vi "Base.vi"(11 "Boolean IN":bool) -> (3 "Boolean OUT":bool)   [LabVIEW 2025]
uses:
  <vilib>/JDP Science/JDP Science Common Utilities/JDP Utility.lvlib
panel:
  in  "Array":void[](array[numeric])
  in  "Multicolumn Listbox":i32(listbox)
  out "XY Graph":cluster{"X":dbl, "Y":dbl}[](graph)
  in  "Tree":string(tree)
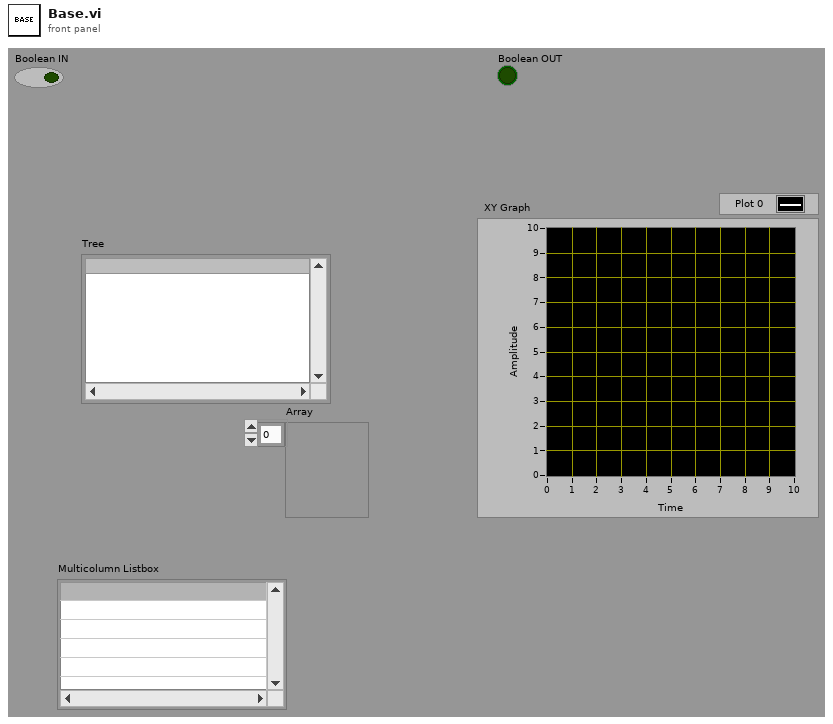
[diagram p1: front panel]
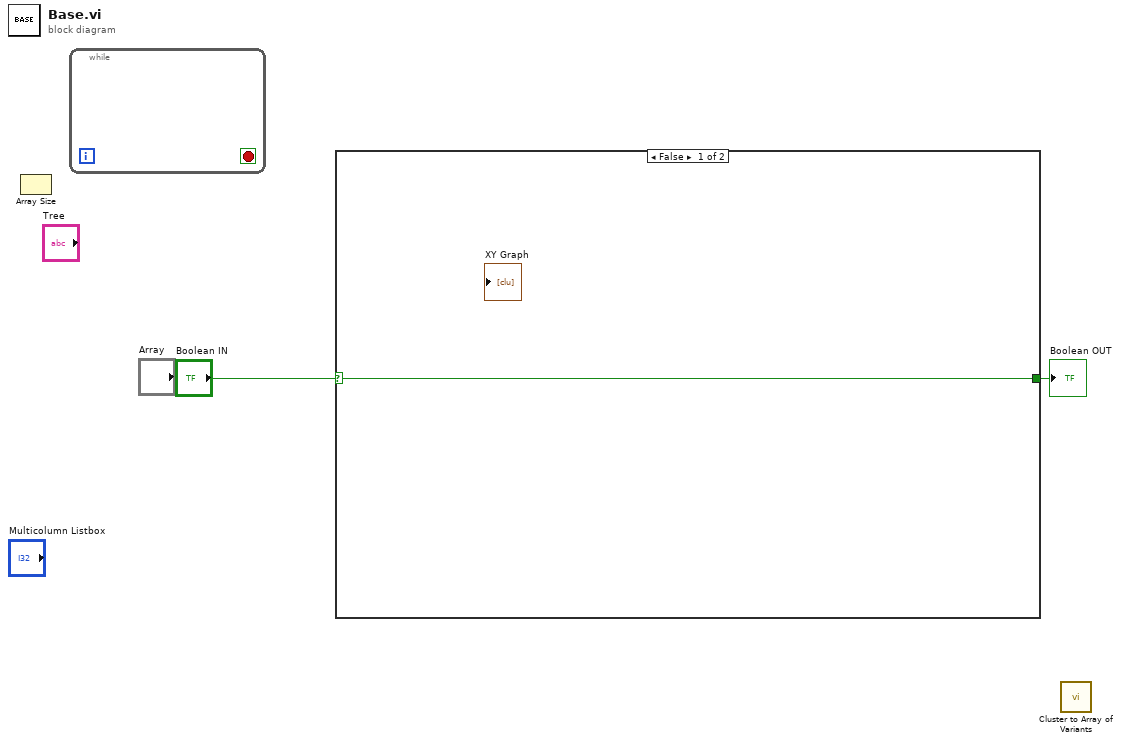
[diagram p0: block diagram]
diagram:
  n1 = Array Size() -> ()  [unwired: 1 in, 1 out]
  n2 = while {
    stop <- _ stop-if-true
  }
  n3 = case shown="False" "Boolean IN" {
    selector: "Boolean IN" -> [w3 w4]
    tunnel: [w3 w4] -> w1
    frame False {
    }
    frame True {
    }
  }
  "Boolean OUT" <- w1
  n4 = call <vilib>:"Cluster to Array of Variants.vi"() -> ()  [unwired: 11 in, 1 out]
